vi "Initialize.vi"(8 "error in (no error)":errorcluster, 11 "Hardware Refs In":T1={"IP Address"="Simulator", "Handle"=0, "Refresh Time (ms)"=0.0}) -> (0 "error out":errorcluster, 3 "Hardware Refs Out":T1={"IP Address"="Simulator", "Handle"=0, "Refresh Time (ms)"=0.0})   [LabVIEW 2013, in "Capacitive.lvlib"]
uses:
  Capacitive.lvlib
  Hardware Configuration.ctl
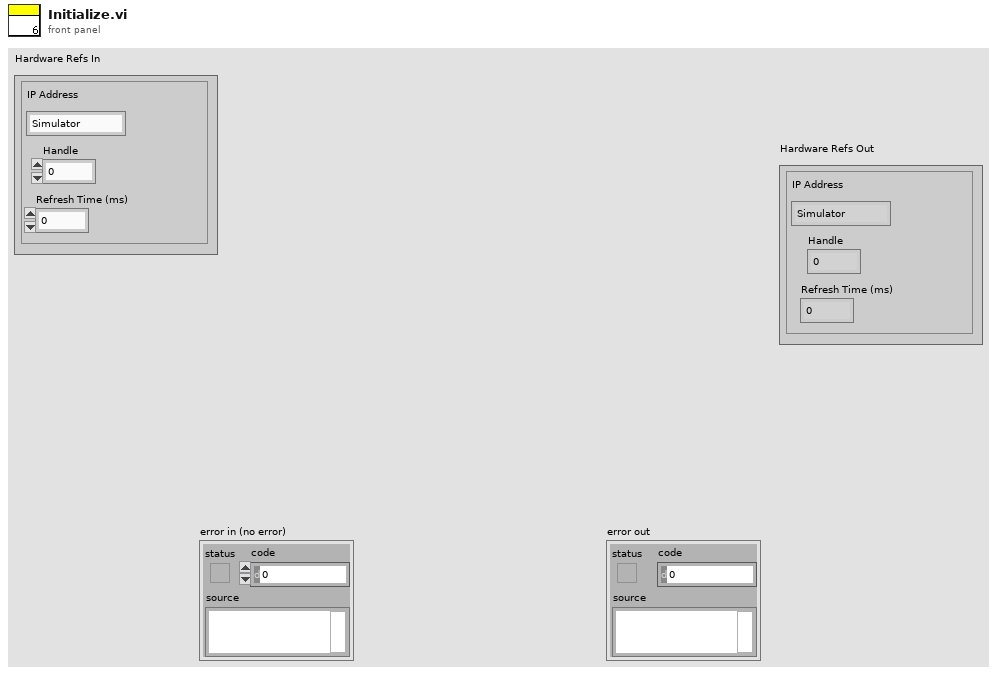
[diagram p1: front panel]
types:
  T1 = typedef "Capacitive.lvlib/Hardware Configuration.ctl" = cluster{"IP Address":string, "Handle":u32, "Refresh Time (ms)":dbl}
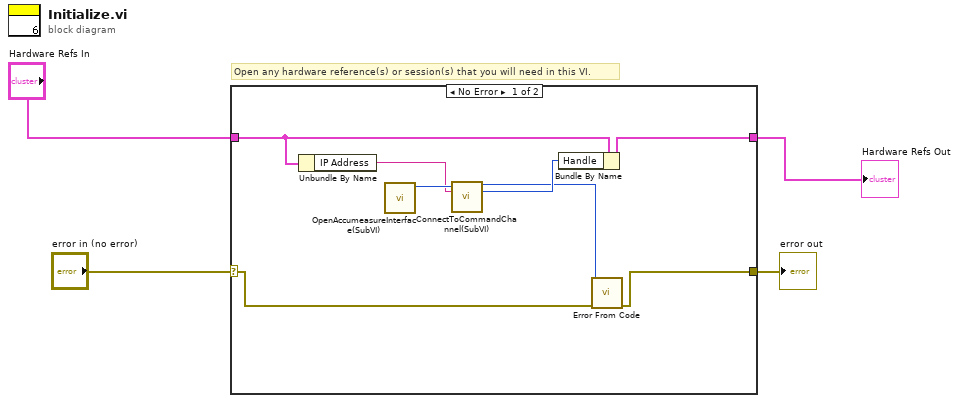
[diagram p0: block diagram]
diagram:
  # "Open any hardware reference(s) or session(s) that you will need in this VI."
  n1 = case shown="No Error" "error in (no error)" {
    selector: "error in (no error)" -> [w7 w13]
    tunnel: [w6 w13] -> w3
    tunnel: "Hardware Refs In" -> [w10 w14]
    tunnel: [w12 w14] -> w1
    frame No Error {
      n2 = Unbundle By Name(w10) -> ("IP Address"=w9:string)
      n3 = call "OpenAccumeasureInterface(SubVI).vi"() -> ("Handle"=w11:u32)  [unwired: 11 in]
      n4 = call "ConnectToCommandChannel(SubVI).vi"("Handle"=w11, "IP Address"=w9) -> ("Status"=w5:i32, "Handle"=w8:u32)  [unwired: 11 in, 1 out]
      n5 = Bundle By Name(cluster=w10, "Handle"=w8) -> (w12:T1)
      n6 = call "Error From Code.vi"("error in (no error)"=w7, "ErrorCode"=w5) -> ("error out"=w6:errorcluster)  [unwired: 9 in]
    }
    frame Error {
    }
  }
  "error out" <- w3
  "Hardware Refs Out" <- w1
